vi "Unary helloworld_Greeter_SayHello.vi"(8 "error in":errorcluster, 10 "Request Data":T2, 11 "gRPC ID":T3) -> (0 "error out":errorcluster, 2 "Response Data":T1, 3 "gRPC ID out":T3)   [LabVIEW 2019, in "helloworld_client.lvlib"]
uses:
  helloworld_client.lvlib
  <vilib>/gRPC/LabVIEW gRPC Library/Server API/typeDefs/grpcId.ctl
  RPC Messages/helloworld_HelloRequest.ctl
  RPC Messages/helloworld_HelloReply.ctl
  3477ff3c-ac1a-41b2-98e0-1f89dff8fa77.vi
  <vilib>/gRPC/LabVIEW gRPC Library/Server API/Server/Get Server DLL Path.vi
  <vilib>/gRPC/LabVIEW gRPC Library/gprc-lvsupport-release.lvlib
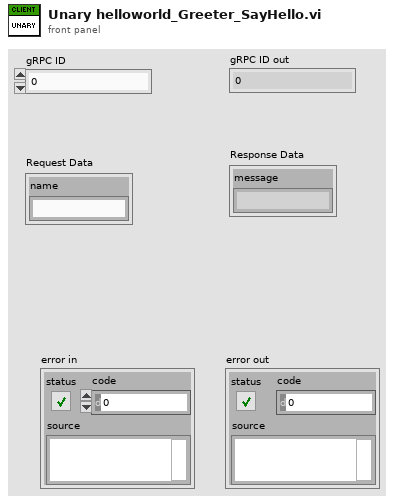
[diagram p1: front panel]
types:
  T1 = typedef "helloworld_client.lvlib/helloworld_HelloReply.ctl" = cluster{"message":string}
  T2 = typedef "helloworld_client.lvlib/helloworld_HelloRequest.ctl" = cluster{"name":string}
  T3 = typedef "gprc-lvsupport-release.lvlib/grpcId.ctl" = u64
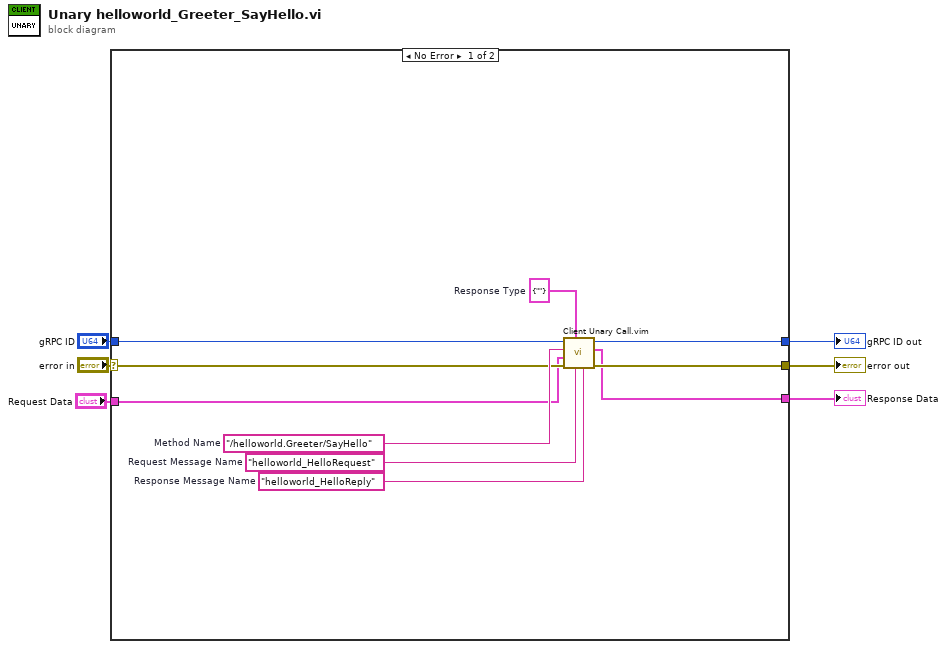
[diagram p0: block diagram]
diagram:
  n1 = case shown="No Error" "error in" {
    selector: "error in" -> [w12 w17]
    tunnel: [w11 w17] -> w5
    tunnel: "gRPC ID" -> [w10 w18]
    tunnel: [w9 w18] -> w3
    tunnel: "Request Data" -> [w8 _]
    tunnel: [w7 _] -> w1
    frame No Error {
      w13 = "helloworld_HelloReply"  # Response Message Name
      w14 = "helloworld_HelloRequest"  # Request Message Name
      w15 = T1 {"message"=""}  # Response Type
      w16 = "/helloworld.Greeter/SayHello"  # Method Name
      n2 = call "Client Unary Call.vim"("Response Message Name"=w13, "Request Message Name"=w14, "Response Type"=w15, "error in (no error)"=w12, "Request Data"=w8, "Method Name"=w16, "Client Ref"=w10) -> ("error out"=w11:errorcluster, "Response Data"=w7:T1, "Client Ref Out"=w9:u64)  [unwired: 2 in]
    }
    frame Error {
    }
  }
  "error out" <- w5
  "gRPC ID out" <- w3
  "Response Data" <- w1
